vi "Unit Test.vi"() -> ()   [LabVIEW 2018]
uses:
  builds/Power_Supply.lvlibp/Custom Control/Channel List.ctl
  builds/Power_Supply.lvlibp/Power Supply.lvclass
  builds/Power_Supply.lvlibp
panel:
  in  "Set Voltage":dbl
  in  "stop":bool
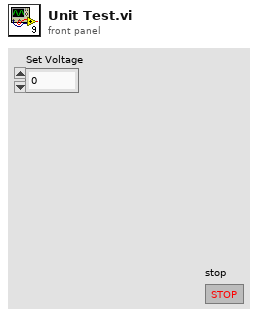
[diagram p1: front panel]
types:
  T1 = typedef "Power_Supply.lvlibp/Channel List.ctl" = enum16{"Channel 1", "Channel 2", "Channel 3", "Channel 4"}
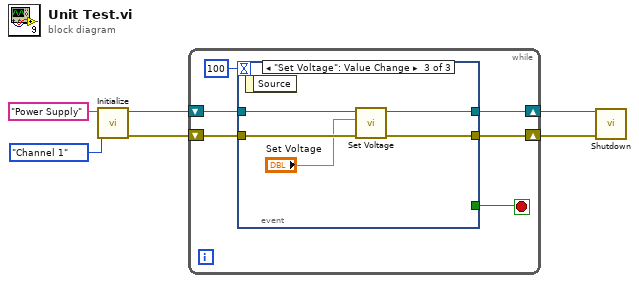
[diagram p0: block diagram]
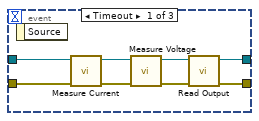
[diagram p2: hidden frame]
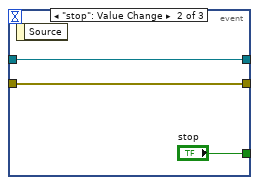
[diagram p3: hidden frame]
diagram:
  n1 = call "Initialize.vi"("Active Channel"=Channel_List."Channel 1", "Device"="Power Supply") -> ("error out"=w5:errorcluster, "Power Supply out"=w6:refnum<class "Power Supply.lvclass">)  [unwired: 8 in]
  n2 = while {
    shift-right: [w8] -> w2
    shift-left: w6 -> [w12]
    shift-right: [w9] -> w1
    shift-left: w5 -> [w11]
    stop <- w7 stop-if-true
    n3 = event shown="[2] \"Set Voltage\": Value Change" {
      selector: _ -> [_ _ _]
      dyn-events: _ -> [_ _ _]
      timeout: 100 -> [_ _ _]
      tunnel: w12 -> [w20 w23 w28]
      tunnel: w11 -> [w19 w22 w26]
      tunnel: [w14 w22 w25] -> w9
      tunnel: [w13 w23 w27] -> w8
      tunnel: [_ "stop" _] -> w7
      event Timeout {
        n4 = event-data() -> ()  [unwired: 1 in, 1 out]
        n5 = call-dynamic "Measure Current.vi"("error in (no error)"=w19, "Power Supply in"=w20) -> ("error out"=w18:errorcluster, "Power Supply out"=w17:refnum<class "Power Supply.lvclass">)  [unwired: 7 in, 1 out]
        n6 = call-dynamic "Measure Voltage.vi"("error in (no error)"=w18, "Power Supply in"=w17) -> ("error out"=w15:errorcluster, "Power Supply out"=w16:refnum<class "Power Supply.lvclass">)  [unwired: 7 in, 1 out]
        n7 = call-dynamic "Read Output.vi"("error in"=w15, "Power Supply in"=w16) -> ("error out"=w14:errorcluster, "Power Supply out"=w13:refnum<class "Power Supply.lvclass">)  [unwired: 7 in, 1 out]
      }
      event "stop": Value Change {
        n8 = event-data() -> ()  [unwired: 1 in, 1 out]
      }
      event "Set Voltage": Value Change {
        n9 = event-data() -> ()  [unwired: 1 in, 1 out]
        n10 = call "Set Voltage.vi"("error in"=w26, "Voltage"="Set Voltage", "Power Supply in"=w28) -> ("error out"=w25:errorcluster, "Power Supply out"=w27:refnum<class "Power Supply.lvclass">)  [unwired: 7 in]
      }
    }
  }
  n11 = call "Shutdown.vi"("error in"=w1, "Power Supply in"=w2) -> ()  [unwired: 8 in, 2 out]
